vi "Config Drive Pipeline Command_wrapper.vi"() -> ()   [LabVIEW 2020]
uses:
  <vilib>/Rock Robotics/WPI/Framework/Command Status Info.ctl
  <vilib>/Rock Robotics/WPI/Framework/Completion Status.ctl
  <vilib>/Rock Robotics/WPI/Framework/Completion Notifier.ctl
panel:
  out "Command Info Out":T1
  in  "Command Info In":T1
  in  "Drive Conditions":T4
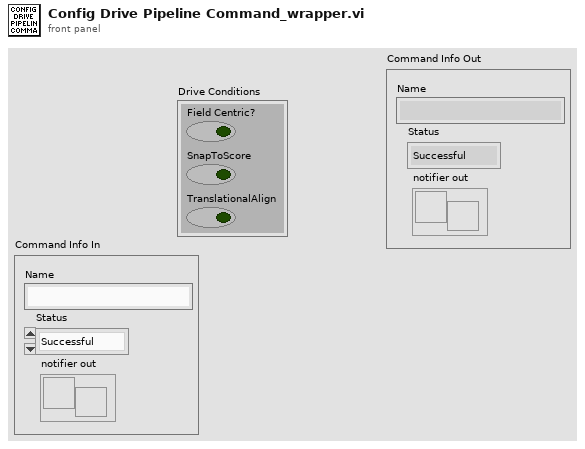
[diagram p1: front panel]
types:
  T1 = typedef "Command Status Info.ctl" = cluster{"Name":string, "Status":T2, "notifier out":T3}
  T2 = typedef "Completion Status.ctl" = enum16{"Successful", "Aborted", "Incomplete"}
  T3 = typedef "Completion Notifier.ctl" = refnum<notifier>
  T4 = cluster{"Field Centric?":bool, "SnapToScore":bool, "TranslationalAlign":bool}
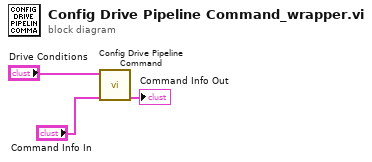
[diagram p0: block diagram]
diagram:
  n1 = call "Config Drive Pipeline Command.vi"("Command Info In"="Command Info In", "Drive Conditions"="Drive Conditions") -> ("Command Info Out"=→"Command Info Out":T1)  [unwired: 9 in]
